vi "Simulation and Arm.vi"(9 "L 2":dbl(slide)=77.0 scale=0.0..200.0, 10 "L 1":dbl(slide)=77.0 scale=0.0..200.0) -> ()   [LabVIEW 2024]
uses:
  GitHub/ME121-25/LabVIEW/SerialVIs/subs/portX.xctl
panel:
  in  "write buffer":string="m.rotate_to_angle(0,0,0)"
  out "resulting string":string
  in  "end effector":cluster{dbl, dbl}={0.0, 154.0} {"?" scale=-200.0..200.0; "?" scale=0.0..200.0}
  out "Angle 3":dbl(knob)=-90.24225061853012 scale=-90.0..90.0
  out "Angle 2":dbl(knob)=-90.24225061853012 scale=-90.0..90.0
  out "Angle 1":dbl(knob)=42.054620502414885 scale=-90.0..90.0
  in  "L 3":dbl(slide)=10.0 scale=0.0..200.0
  in  "?":refnum<visa-resource-name>(xcontrol)
  out "2D Picture":picture
  out "XY Graph":cluster{"X":dbl, "Y":dbl}[](graph)
  # "Come use my 3DOF robot arm! You can make the LEGO minifigure go wherever you wish without it falling off its chair (as long as it is within reason)!\n\n1) Make sure you are connected to the ESP32 by choosing the correct port\n2) Ensure that the arm lengths of the arm are correct \n2) Check out the workable area of my arm. You are allowed to go whenever you want within that space.\n3) Enter the (x,y) coordinate \n2) Press run and see what happens"
  # "1)"
  # "4)"
  # "2)"
  # "3)"
  # "3)"
  # "x"
  # "y"
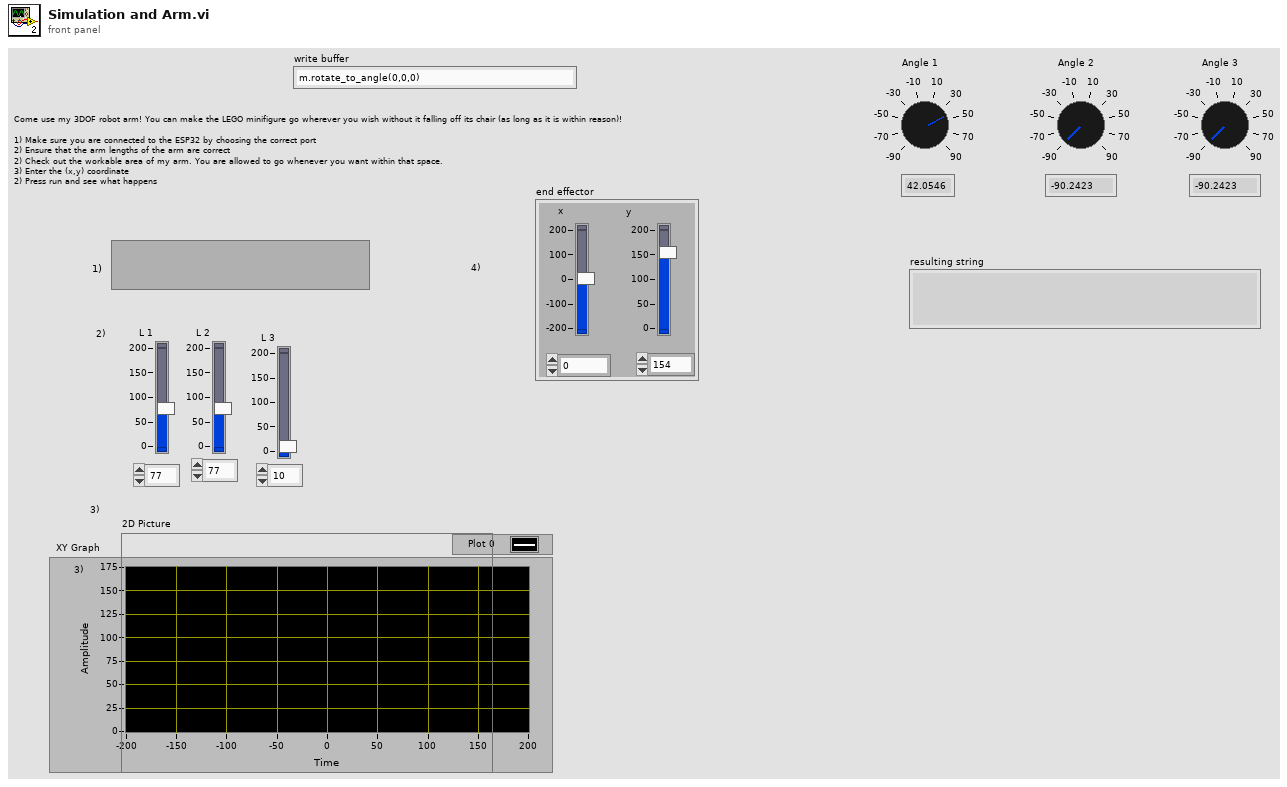
[diagram p1: front panel]
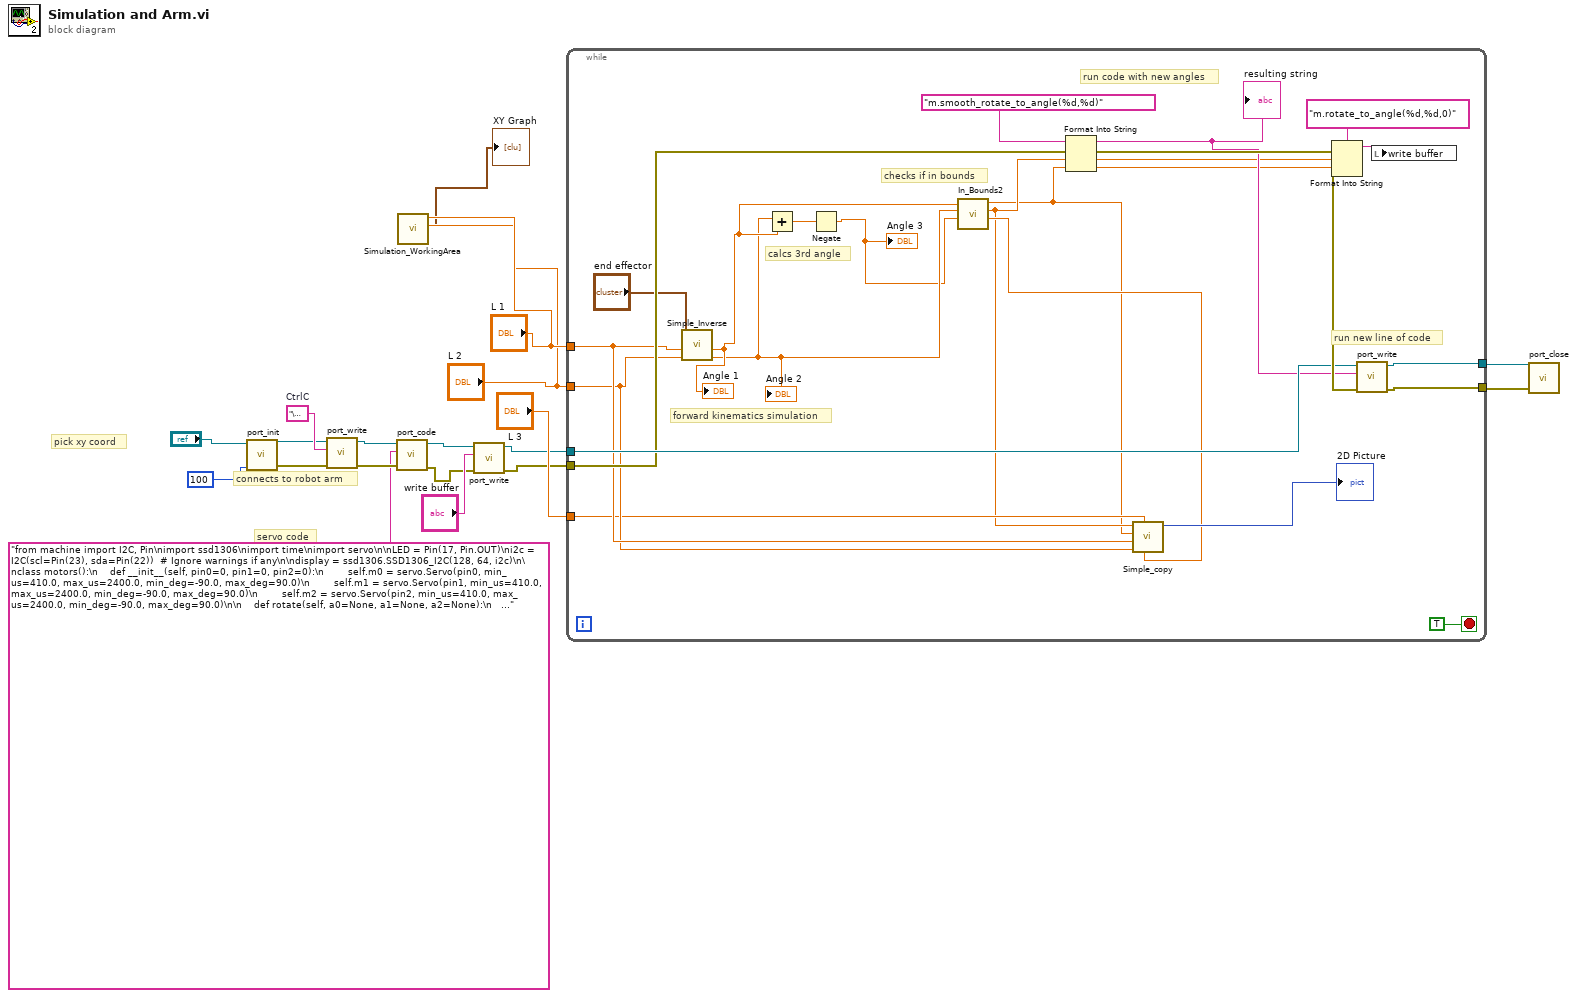
[diagram p0: block diagram]
diagram:
  w19 = "\u0003"  # CtrlC
  # "pick xy coord"
  # "servo code"
  # "connects to robot arm"
  n1 = call "port_init.vi"("Timeout (ms)"=u32 100, "VISA Refnum in"="?") -> ("error out"=w17:errorcluster, "VISA Refnum out"=w18:refnum<visa-resource-name>)  [unwired: 8 in]
  n2 = call "port_write.vi"("error in (no error)"=w17, "write buffer"=w19, "VISA Refnum in"=w18) -> ("error out"=w14:errorcluster, "VISA Refnum out"=w15:refnum<visa-resource-name>)  [unwired: 7 in]
  n3 = call "port_code.vi"("error in (no error)"=w14, "Code to run"="from machine import I2C, Pin\nimport ssd1306\nimport time\nimport servo\n\nLED = Pin(17, Pin.OUT)\ni2c = I2C(scl=Pin(23), sda=Pin(22))  # Ignore warnings if any\n\ndisplay = ssd1306.SSD1306_I2C(128, 64, i2c)\n\nclass motors():\n    def __init__(self, pin0=0, pin1=0, pin2=0):\n        self.m0 = servo.Servo(pin0, min_us=410.0, max_us=2400.0, min_deg=-90.0, max_deg=90.0)\n        self.m1 = servo.Servo(pin1, min_us=410.0, max_us=2400.0, min_deg=-90.0, max_deg=90.0)\n        self.m2 = servo.Servo(pin2, min_us=410.0, max_us=2400.0, min_deg=-90.0, max_deg=90.0)\n\n    def rotate(self, a0=None, a1=None, a2=None):\n        if a0 is not None:\n            self.m0.write(a0)\n        if a1 is not None:\n            self.m1.write(a1)\n        if a2 is not None:\n            self.m2.write(a2)\n        self.show()\n\n    def show(self):\n        display.fill(0)\n        display.text('Motors at:', 0, 0, 1)\n        display.text(f'%d, %d, %d' % (self.m0.read(), self.m1.read(), self.m2.read()), 0, 12, 1)\n        display.show()\n\n    def read(self):\n        # Return the current angles of the motors\n        return self.m0.read(), self.m1.read(), self.m2.read()\n\n    def rotate_to_angle(self, angle1, angle2, angle3):\n        # Directly set motors to the target angle\n        self.rotate(angle1, angle2, angle3)\n        #time.sleep(1)  # Add some delay to let the motors move\n\n    def smooth_rotate_to_angle(self, target1, target2, increments=50, delay=0.4):\n        if increments <= 0:  # Prevent division by zero\n            increments = 10  # Default to at least one step\n        # Get current motor positions\n        current1, current2, current3 = self.read()\n\n        # Compute step sizes for smooth transitions\n        step1 = (target1 - current1) / increments\n        step2 = (target2 - current2) / increments\n\n        # Incrementally update angles to the target positions\n        for i in range(increments):\n            new1 = current1 + step1 * (i + 1)\n            new2 = current2 + step2 * (i + 1)\n\n            # Ensure angles stay within the valid range\n            new1 = max(-90, min(90, new1))\n            new2 = max(-90, min(90, new2))\n\n            # Calculate new3 as the inverse sum of new1 and new2\n            new3 = -(new1 + new2)\n\n            # Ensure new3 stays within the valid range\n            new3 = max(-90, min(90, new3))\n\n            # Apply the new angles to the motors\n            self.rotate(new1, new2, new3)\n            time.sleep(delay)  # Add delay to control the speed of movement\n\n\n# Initialize motor controller\nm = motors(0, 1, 2)\n#m.smooth_rotate_to_angle(90,0,0)\n\n\n\n", "VISA Refnum in"=w15) -> ("error out"=w3:errorcluster, "VISA Refnum out"=w4:refnum<visa-resource-name>)  [unwired: 7 in]
  n4 = call "Simulation_WorkingArea.vi"("L 2"="L 2", "L 1"="L 1") -> ("XY Graph 2"=→"XY Graph":cluster{"X":dbl, "Y":dbl}[])  [unwired: 7 in, 2 out]
  n5 = call "port_write.vi"("error in (no error)"=w3, "write buffer"="write buffer", "VISA Refnum in"=w4) -> ("error out"=w1:errorcluster, "VISA Refnum out"=w2:refnum<visa-resource-name>)  [unwired: 7 in]
  n6 = while {
    tunnel: "L 1" -> [w33]
    tunnel: "L 2" -> [w32]
    tunnel: w2 -> [w39]
    tunnel: [w38] -> w12
    tunnel: [w37] -> w11
    tunnel: w1 -> [w36]
    tunnel: "L 3" -> [w31]
    stop <- TRUE stop-if-true
    # "run new line of code"
    # "checks if in bounds"
    # "run code with new angles"
    # "calcs 3rd angle"
    # "forward kinematics simulation"
    n7 = call "Simple_Inverse.vi"("L 2"=w32, "L 1"=w33, "end effector"="end effector") -> ("Angle 2"=w29:dbl, "Angle1"=w30:dbl)  [unwired: 7 in]
    "Angle 1" <- w30
    "Angle 2" <- w29
    n8 = Add(x=w30, y=w29) -> (x+y=w35:dbl)
    n9 = Negate(x=w35) -> (-x=w28:dbl)
    "Angle 3" <- w28
    n10 = call "In_Bounds2.vi"("Angle in 3"=w28, "Angle in 2"=w29, "Angle in"=w30) -> ("angle 3"=w27:dbl, "angle 1"=w21:dbl, "angle 2"=w20:dbl)  [unwired: 6 in]
    n11 = Format Into String "Format Into String"(format string="m.smooth_rotate_to_angle(%d,%d)", error in=w36, w21, w20) -> (resulting string=w24:string, error out=w40:errorcluster)  [unwired: 1 in]
    "resulting string" <- w24
    n12 = call "Simple_copy.vi"("Angle 3"=w27, "L 3"=w31, "L 2"=w32, "L 1"=w33, "Angle 2"=w20, "Angle1"=w21) -> ("2D Picture"=→"2D Picture":picture)  [unwired: 3 in, 2 out]
    n13 = Format Into String "Format Into String"(format string="m.rotate_to_angle(%d,%d,0)", w21, w20) -> (resulting string=w22:string)  [unwired: 2 in, 1 out]
    n14 = call "port_write.vi"("error in (no error)"=w40, "write buffer"=w24, "VISA Refnum in"=w39) -> ("error out"=w37:errorcluster, "VISA Refnum out"=w38:refnum<visa-resource-name>)  [unwired: 7 in]
    n15 = local write "write buffer"(w22) -> ()
  }
  n16 = call "port_close.vi"("error in (no error)"=w11, "VISA Refnum in"=w12) -> ()  [unwired: 10 in]
